vi "Rising Edge Detector with Data Valid.vi"(9 "Data Valid":bool, 10 "signal":bool) -> (2 "edge detected":bool)   [LabVIEW 2012]
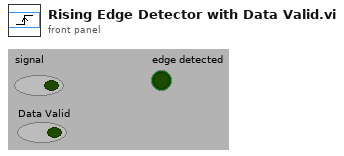
[diagram p1: front panel]
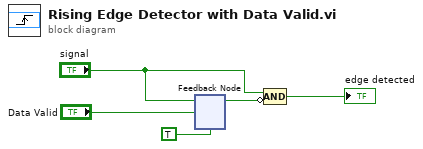
[diagram p0: block diagram]
diagram:
  n1 = feedback-in #1("signal", "Data Valid") -> ()
  n2 = feedback #1(TRUE) -> (w4:bool)
  n3 = Compound Arithmetic op=AND("signal", invert w4) -> (→"edge detected":bool)
